vi "_Initialize.vi"(7 "Refs":T2, 9 "Action in":T1 caption="Action", 10 "Display State In in":T3 caption="State", 11 "Data In in":T6) -> (1 "Action out":T1 caption="Action", 2 "Display State In out":T3 caption="State", 3 "Data In out":T6)   [LabVIEW 2013, in "UI_TimeSelector.xctl"]
uses:
  UI_TimeSelector.xctl
  Data.ctl
  State.ctl
  Typedefs/INTERNAL-DATA.ctl
  Interface/DEF-Mode.ctl
  Typedefs/INTERNAL-REFs.ctl
  <vilib>/_xctls/Action.ctl
  <vilib>/_xctls/XControlSupport.lvlib
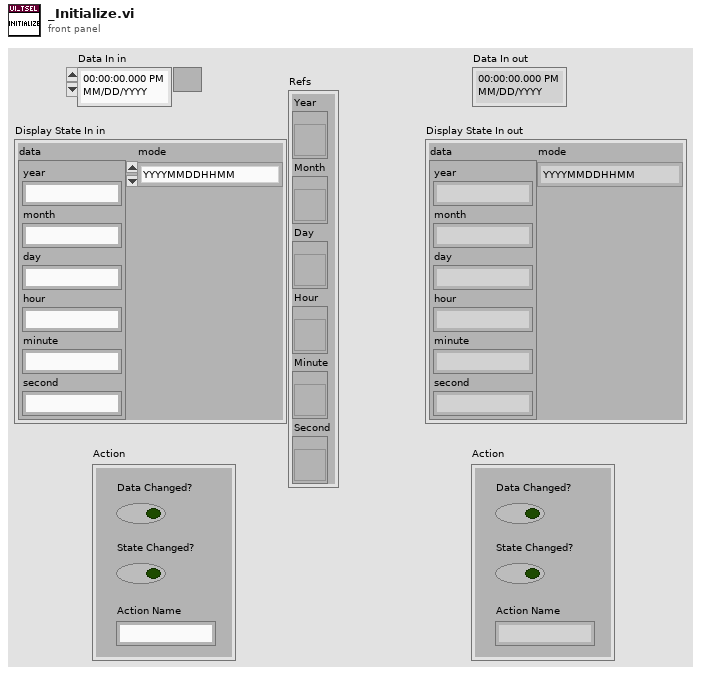
[diagram p1: front panel]
types:
  T1 = typedef "XControlSupport.lvlib/Action.ctl" = cluster{"Data Changed?":bool, "State Changed?":bool, "Action Name":string}
  T2 = typedef "UI_TimeSelector.xctl/INTERNAL-REFs.ctl" = cluster{"Year":refnum<vi>, "Month":refnum<vi>, "Day":refnum<vi>, "Hour":refnum<vi>, "Minute":refnum<vi>, "Second":refnum<vi>}
  T3 = typedef "UI_TimeSelector.xctl/State.ctl" = cluster{"data":T4, "mode":T5}
  T4 = typedef "UI_TimeSelector.xctl/INTERNAL-DATA.ctl" = cluster{"year":string, "month":string, "day":string, "hour":string, "minute":string, "second":string}
  T5 = typedef "UI_TimeSelector.xctl/DEF-Mode.ctl" = enum16{"YYYYMMDDHHMM", "YYYYMMDDHHMMSS", "YYYY", "YYYYMM", "YYYYMMDD", "HHMM", "HHMMSS"}
  T6 = typedef "UI_TimeSelector.xctl/Data.ctl" = timestamp
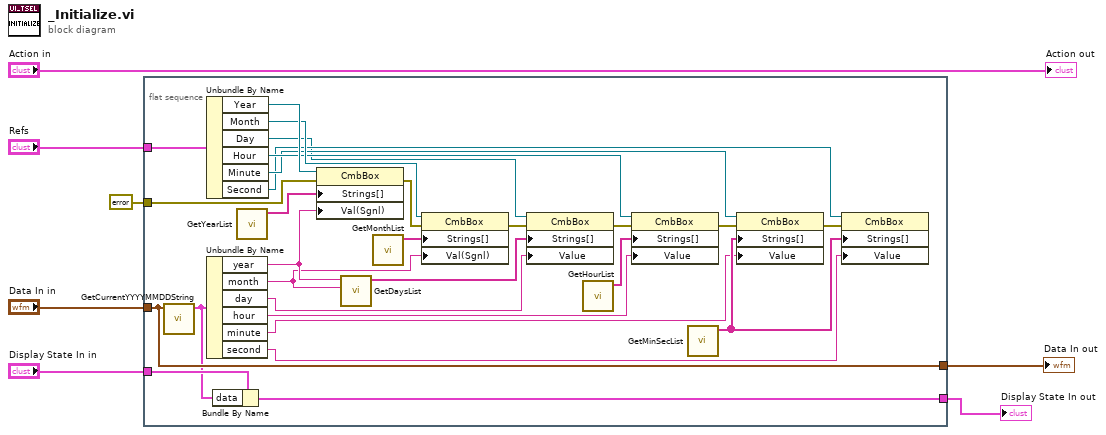
[diagram p0: block diagram]
diagram:
  n1 = flat-sequence {
    tunnel: "Display State In in" -> [w35]
    tunnel: [w9] -> w5
    tunnel: "Data In in" -> [w22]
    tunnel: [w22] -> w7
    tunnel: "Refs" -> [w23]
    tunnel: errorcluster {"status"=FALSE, "code"=0, "source"=""} ("error in (no error)") -> [w21]
    frame #0 {
      n2 = call "GetCurrentYYYYMMDDString.vi"("displayTime"=w22) -> ("data"=w8:T4)  [unwired: 10 in]
      n3 = Unbundle By Name(w23) -> ("Year"=w34:refnum<vi>, "Month"=w33:refnum<vi>, "Day"=w16:refnum<vi>, "Hour"=w30:refnum<vi>, "Minute"=w29:refnum<vi>, "Second"=w28:refnum<vi>)
      n4 = Unbundle By Name(w8) -> ("year"=w19:string, "month"=w18:string, "day"=w14:string, "hour"=w12:string, "minute"=w11:string, "second"=w10:string)
      n5 = Bundle By Name(cluster=w35, "data"=w8) -> (w9:T3)
      n6 = call "GetYearList.vi"() -> ("Array"=w27:string[])  [unwired: 11 in]
      n7 = property class="CmbBox"(reference=w34, error in=w21, "Strings[]"=w27, "Val(Sgnl)"=w19) -> (error out=w20:errorcluster)  [unwired: 1 out]
      n8 = call "GetDaysList.vi"("month"=w18, "year"=w19) -> ("Array"=w17:string[])  [unwired: 9 in]
      n9 = call "GetMonthList.vi"() -> ("Moth List"=w26:string[])  [unwired: 11 in]
      n10 = property class="CmbBox"(reference=w33, error in=w20, "Strings[]"=w26, "Val(Sgnl)"=w18) -> (error out=w15:errorcluster)  [unwired: 1 out]
      n11 = property class="CmbBox"(reference=w16, error in=w15, "Strings[]"=w17, "Value"=w14) -> (error out=w13:errorcluster)  [unwired: 1 out]
      n12 = call "GetHourList.vi"() -> ("Hour List"=w25:string[])  [unwired: 11 in]
      n13 = property class="CmbBox"(reference=w30, error in=w13, "Strings[]"=w25, "Value"=w12) -> (error out=w32:errorcluster)  [unwired: 1 out]
      n14 = call "GetMinSecList.vi"() -> ("Min/Sec List"=w24:string[])  [unwired: 11 in]
      n15 = property class="CmbBox"(reference=w29, error in=w32, "Strings[]"=w24, "Value"=w11) -> (error out=w31:errorcluster)  [unwired: 1 out]
      n16 = property class="CmbBox"(reference=w28, error in=w31, "Strings[]"=w24, "Value"=w10) -> ()  [unwired: 2 out]
    }
  }
  "Data In out" <- w7
  "Display State In out" <- w5
  "Action out" <- "Action in"
